vi "Ready Led Logic.vi"(9 "Stop":bool, 10 "Threshold Temp":bool, 11 "Elapsed Time (s)":dbl) -> (3 "Tea Ready":bool)   [LabVIEW 2022 SP3]
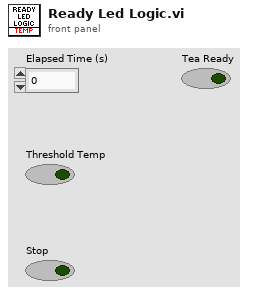
[diagram p1: front panel]
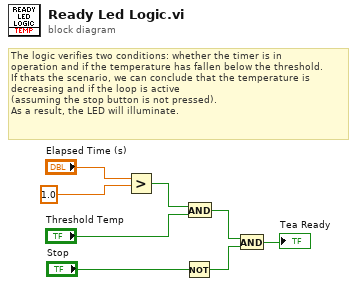
[diagram p0: block diagram]
diagram:
  # "The logic verifies two conditions: whether the timer is in \noperation and if the temperature has fallen below the threshold.\nIf thats the scenario, we can conclude that the temperature is\ndecreasing and if the loop is active \n(assuming the stop button is not pressed). \nAs a result, the LED will illuminate."
  n1 = Greater?(x="Elapsed Time (s)", y=1.0) -> (0:w1:bool)
  n2 = Not(x="Stop") -> (.not. x?=w5:bool)
  n3 = And(x=w1, y="Threshold Temp") -> (x .and. y?=w4:bool)
  n4 = And(x=w4, y=w5) -> (x .and. y?=→"Tea Ready":bool)
